vi "ProducerConsumerEvents.vi"(0 "d1":dbl, 1 "from_right1":i16, 2 "state":i16, 3 "Numeric":i16, 5 "d2":dbl, 7 "reward":i16, 9 "v1":dbl, 11 "v2":dbl, 12 "frome_right2":i16, 13 "ori_action":i16) -> (8 "action":i16, 15 "new_state":i16)   [LabVIEW 2022 SP3]
doc: "Use this template to build a producer/consumer design pattern with events to produce queue items. Use this design pattern instead of the User Interface Event Handler pattern for user interfaces when you want to execute code asynchronously in response to an event without slowing the user interface responsiveness."
panel:
  in  "q":dbl[][](array[numeric])=[[0.0, 0.0, 0.0], [0.0, 0.0, 0.0], [0.0, 0.0, 0.0], [0.0, 0.0, 0.0]]
  in  "stop":bool
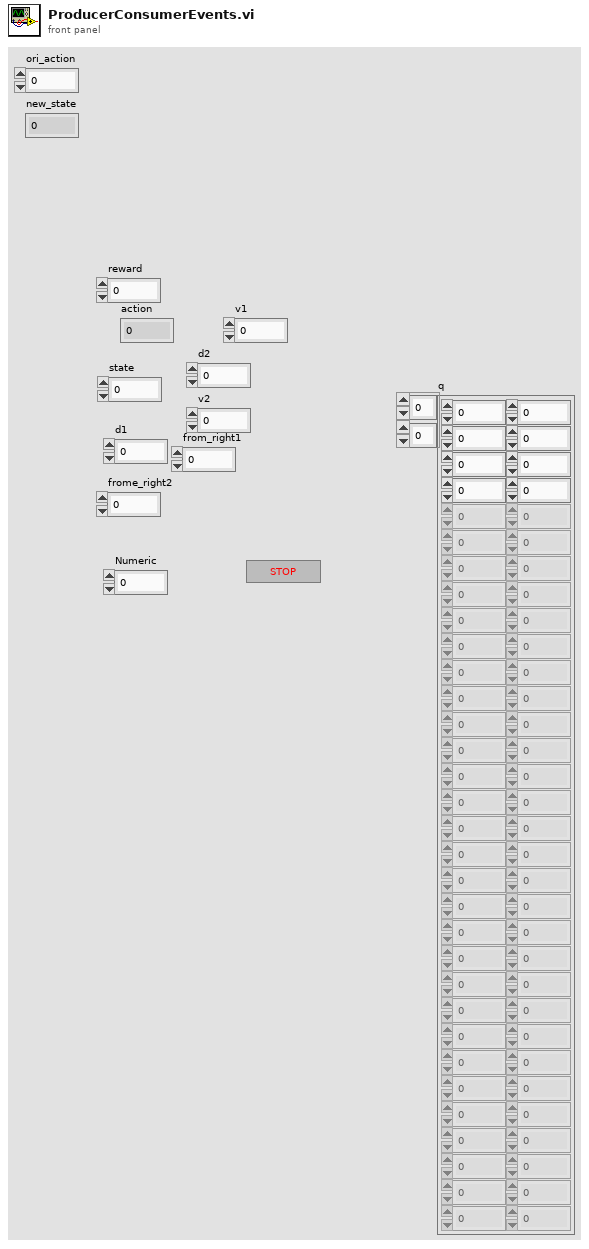
[diagram p1: front panel]
types:
  T1 = cluster{i32, i32, dbl, dbl, dbl, dbl, dbl[][], i32, i32, i32}
  T2 = cluster{"from_right1":i16, "frome_right2":i16, "v1":dbl, "v2":dbl, "d1":dbl, "d2":dbl, "q":dbl[][], "reward":i16, "state":i16, "ori_action":i16}
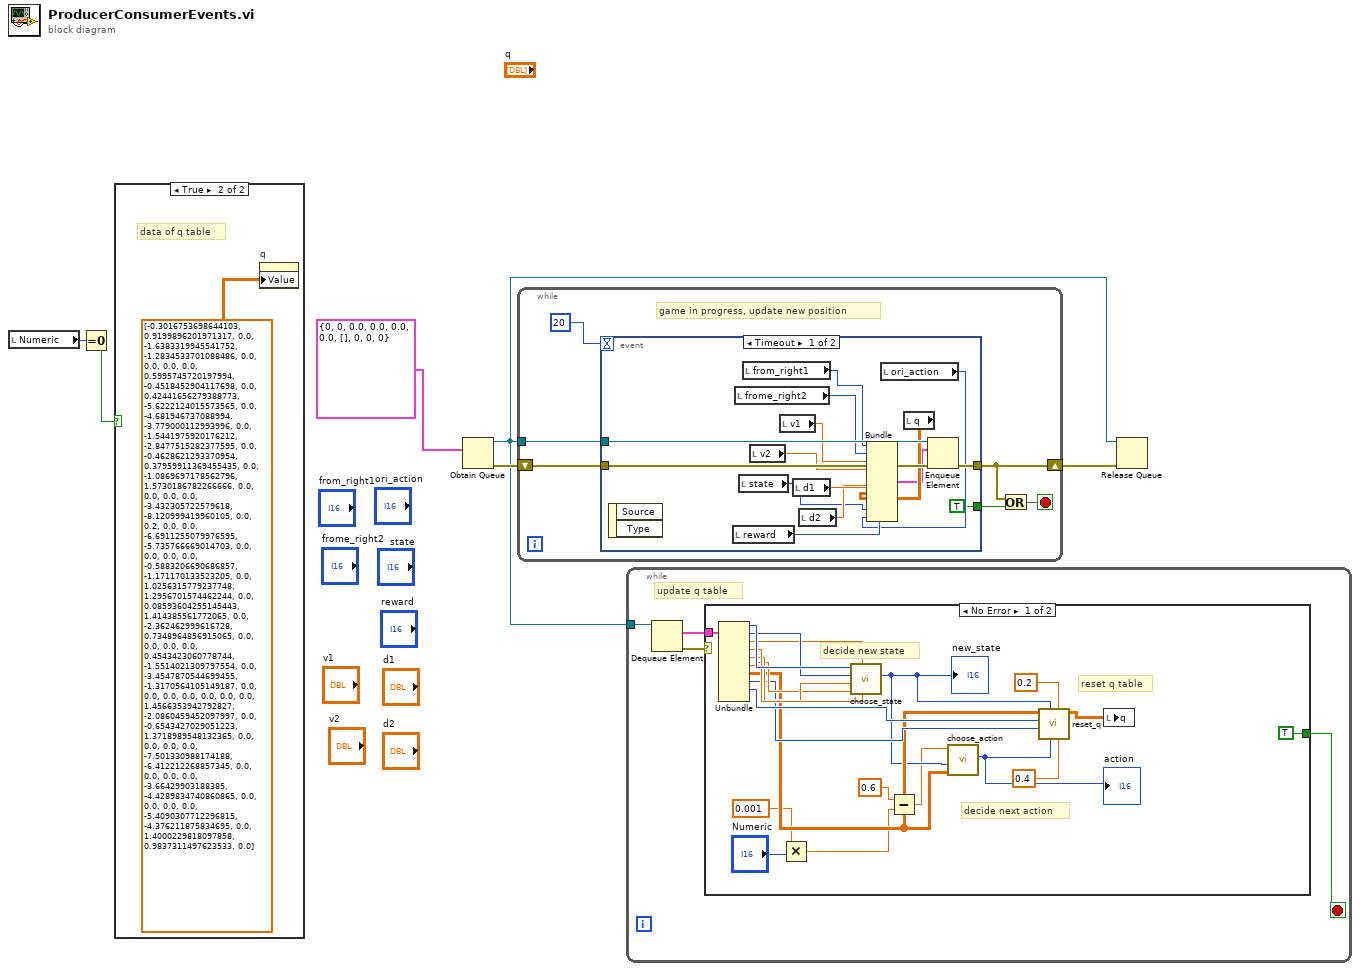
[diagram p0: block diagram]
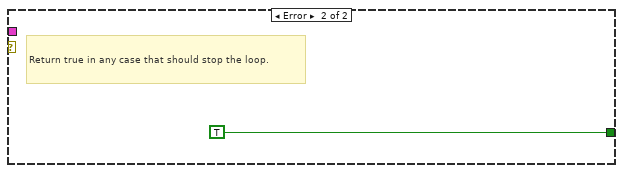
[diagram p3: hidden frame]
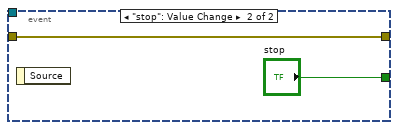
[diagram p4: hidden frame]
diagram:
  n1 = local read "Numeric"() -> (w2:i16)
  n2 = Equal To 0?(x=w2) -> (x = 0?=w1:bool)
  n3 = case shown="True" w1 {
    frame False {
    }
    frame True {
      # "data of q table"
      n4 = property on="q" class="Arr (strict)"("Value"=dbl[][] [[-0.3016753698644103, 0.9199896201971317, 0.0], [-1.6383319945541752, -1.2834533701088486, 0.0], [0.0, 0.0, 0.0], [0.5995745720197994, -0.4518452904117698, 0.0], [0.42441656279388773, -5.6222124015573565, 0.0], [-4.681946737088994, -3.779000112993996, 0.0], [-1.5441975920176212, -2.8477515282377595, 0.0], [-0.4628621293370954, 0.37959911369455435, 0.0], [-1.0869697178562796, 1.5730186782266666, 0.0], [0.0, 0.0, 0.0], [-3.432305722579618, -8.120999419960105, 0.0], [0.2, 0.0, 0.0], [-6.6911255079976595, -5.735766669014703, 0.0], [0.0, 0.0, 0.0], [-0.5883206690686857, -1.171170133523205, 0.0], [1.0256315779237748, 1.2956701574462244, 0.0], [0.08593604255145443, 1.414385561772065, 0.0], [-2.362462999616728, 0.7348964856915065, 0.0], [0.0, 0.0, 0.0], [0.4543423060778744, -1.5514021309797554, 0.0], [-3.4547870544699455, -1.3170564105149187, 0.0], [0.0, 0.0, 0.0], [0.0, 0.0, 0.0], [1.4566353942792827, -2.0860459452097997, 0.0], [-0.6543427029051223, 1.3718989548132365, 0.0], [0.0, 0.0, 0.0], [-7.501330988174188, -6.412212268857345, 0.0], [0.0, 0.0, 0.0], [-3.66429903188385, -4.4289834740860865, 0.0], [0.0, 0.0, 0.0], [-5.4090307712296815, -4.376211875834695, 0.0], [1.4000229818097858, 0.9837311497623533, 0.0]] ("q 2")) -> ()  [unwired: 2 in, 2 out]
    }
  }
  n5 = Obtain Queue(element data type=T1 {0, 0, 0.0, 0.0, 0.0, 0.0, [], 0, 0, 0}) -> (queue out=w4:refnum<queue>, error out=w6:errorcluster)  [unwired: 4 in, 1 out]
  n6 = while {
    shift-right: [w9] -> w5
    shift-left: w6 -> [w12]
    tunnel: w4 -> [w13]
    stop <- w10 stop-if-true
    # "game in progress, update new position"
    n7 = event shown="[0] Timeout" {
      selector: _ -> [_ _]
      dyn-events: _ -> [_ _]
      timeout: 20 -> [_ _]
      tunnel: w13 -> [w28 _]
      tunnel: w12 -> [w27 w29]
      tunnel: [w26 w29] -> w9
      tunnel: [TRUE ("stop") "stop"] -> w11
      event Timeout {
        n8 = event-data() -> ()  [unwired: 1 in, 2 out]
        n9 = local read "reward"() -> (w19:i16)
        n10 = local read "frome_right2"() -> (w24:i16)
        n11 = local read "state"() -> (w18:i16)
        n12 = local read "from_right1"() -> (w25:i16)
        n13 = local read "v2"() -> (w22:dbl)
        n14 = local read "v1"() -> (w23:dbl)
        n15 = local read "d1"() -> (w21:dbl)
        n16 = local read "d2"() -> (w20:dbl)
        n17 = local read "ori_action"() -> (w17:i16)
        n18 = local read "q"() -> (w16:dbl[][])
        n19 = Bundle("from_right1"=w25, "frome_right2"=w24, "v1"=w23, "v2"=w22, "d1"=w21, "d2"=w20, "q"=w16, "reward"=w19, "state"=w18, "ori_action"=w17) -> (w15:T2)  [unwired: 1 in]
        n20 = Enqueue Element(queue=w28, element=w15, error in (no error)=w27) -> (error out=w26:errorcluster)  [unwired: 1 in, 2 out]
      }
      event "stop": Value Change {
        n21 = event-data() -> ()  [unwired: 1 in, 1 out]
      }
    }
    n22 = Or(x=w9, y=w11) -> (x .or. y?=w10:bool)
  }
  n23 = while {
    tunnel: w4 -> [w34]
    stop <- w31 stop-if-true
    # "update q table"
    n24 = Dequeue Element(queue=w34) -> (element=w32:T1, error out=w33:errorcluster)  [unwired: 2 in, 2 out]
    n25 = case shown="No Error" w33 {
      tunnel: w32 -> [w55 _]
      tunnel: [TRUE TRUE] -> w31
      frame No Error {
        # "decide next action"
        # "reset q table"
        # "decide new state"
        n26 = Unbundle(w55) -> (w54:i32, w53:i32, w52:dbl, w51:dbl, w50:dbl, w49:dbl, w46:dbl[][], w47:i32, w48:i32)  [unwired: 1 out]
        n27 = Multiply(x=0.001, y="Numeric") -> (x*y=w37:dbl)
        n28 = call "choose_state.vi"("v2"=w51, "v1"=w52, "d2"=w49, "d1"=w50, "from_right2"=w53, "from_right1"=w54) -> ("state"=w41:i16)  [unwired: 5 in]
        "new_state" <- w41
        n29 = Subtract(x=0.6, y=w37) -> (x-y=w35:dbl)
        n30 = call "choose_action.vi"("Q"=w46, "state"=w41, "epson"=w35) -> ("action"=w36:u8)  [unwired: 8 in]
        "action" <- w36
        n31 = call "reset_q.vi"("discountfactor"=0.4, "learningrate"=0.2, "new state"=w41, "Numeric"=w36, "reward"=w47, "state"=w48, "Q in"=w46) -> ("Q out"=w43:dbl[][])  [unwired: 4 in]
        n32 = local write "q"(w43) -> ()
      }
      frame Error {
        # "Return true in any case that should stop the loop."
      }
    }
  }
  n33 = Release Queue(queue=w4, error in (no error)=w5) -> ()  [unwired: 1 in, 3 out]
